vi "Dátumformátomú szöveg átalakítása.vi"(10 "Szöveg, amiben keresni kell":string) -> (3 "Dátum értéke számban":dbl)   [LabVIEW 2014]
doc: "Ez a SubVI átalakítja a dátum formátumú szöveget szám értékké. \nEgy szövegben megkeresi a dátum formátumú szöveget és átalakítja dátum formátumú adattá.\nEzután a dátum formátumú adat átalakul double formátumú számmá."
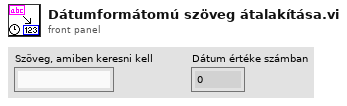
[diagram p1: front panel]
types:
  T1 = typedef "LVDateTimeRec.ctl" = cluster{"fractional second":dbl, "second":i32, "minute":i32, "hour":i32, "day of month":i32, "month":i32, "year":i32, "day of week":i32, "day of year":i32, "DST":i32}
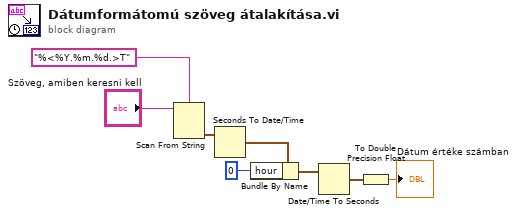
[diagram p0: block diagram]
diagram:
  n1 = Scan From String(format string="%<%Y.%m.%d.>T", input string="Szöveg, amiben keresni kell") -> (output 1=w6:timestamp)  [unwired: 3 in, 3 out]
  n2 = Seconds To Date/Time(time stamp (now)=w6) -> (date time rec=w5:T1)  [unwired: 1 in]
  n3 = Bundle By Name(cluster=w5, "hour"=0) -> (w3:T1)
  n4 = Date/Time To Seconds(2:w3) -> (0:w2:timestamp)  [unwired: 1 in]
  n5 = To Double Precision Float(number=w2) -> (double precision float=→"Dátum értéke számban":dbl)
